vi "Bundles.vi"() -> ()   [LabVIEW 2022 SP3]
panel:
  out "String 2":string
  out "Boolean 2":bool
  out "Numeric 2":dbl
  in  "String":string
  in  "Boolean":bool
  in  "Numeric":dbl
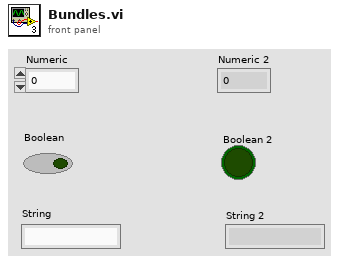
[diagram p1: front panel]
types:
  T1 = cluster{"Numeric":dbl, "Boolean":bool, "String":string}
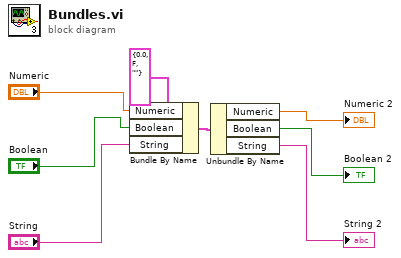
[diagram p0: block diagram]
diagram:
  n1 = Bundle By Name "Bundle By Name"(cluster=T1 {"Numeric"=0.0, "Boolean"=FALSE, "String"=""}, "Numeric"="Numeric", "Boolean"="Boolean", "String"="String") -> (w4:T1)
  n2 = Unbundle By Name "Unbundle By Name"(w4) -> ("Numeric"=→"Numeric 2":dbl, "Boolean"=→"Boolean 2":bool, "String"=→"String 2":string)
